vi "Set Server State UE.vi"(10 "Server State UE":refnum<user-event>, 11 "Template Server in":refnum<class "HVC3.lvclass">) -> (3 "Template Server out":refnum<class "HVC3.lvclass">)   [LabVIEW 2019, in "HVC3.lvlib" / "HVC3.lvclass"]
uses:
  HVC3.lvclass
  typeDefs/Server State Data.ctl
  HVC3.lvclass/HVC3.ctl
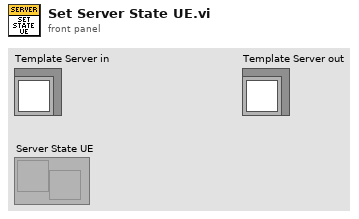
[diagram p1: front panel]
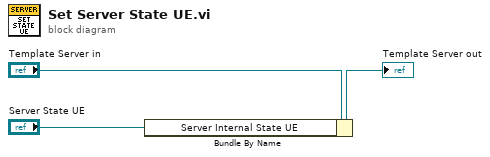
[diagram p0: block diagram]
diagram:
  n1 = Bundle By Name(cluster="Template Server in", "Server Internal State UE"="Server State UE") -> (→"Template Server out":refnum<class "HVC3.lvclass">)
